vi "TLA_Picking List Get Table.vi"(8 "error in (no error)":errorcluster caption="错误输入（无错误）", 10 "JobNo":string, 11 "Traceability 引用句柄":refnum<k24>) -> (0 "error out":errorcluster caption="错误输出", 2 ".NET:System.Data.DataTable":T1 {"RemotingFormat" items=["Xml", "Binary"]}, 3 "Traceability 引用句柄输出":refnum<k24>)   [LabVIEW 2014, in "Traceability.lvlib"]
uses:
  D:/webservice/Traceability.dll
  Traceability.dll
  System.Data
  Traceability.lvlib
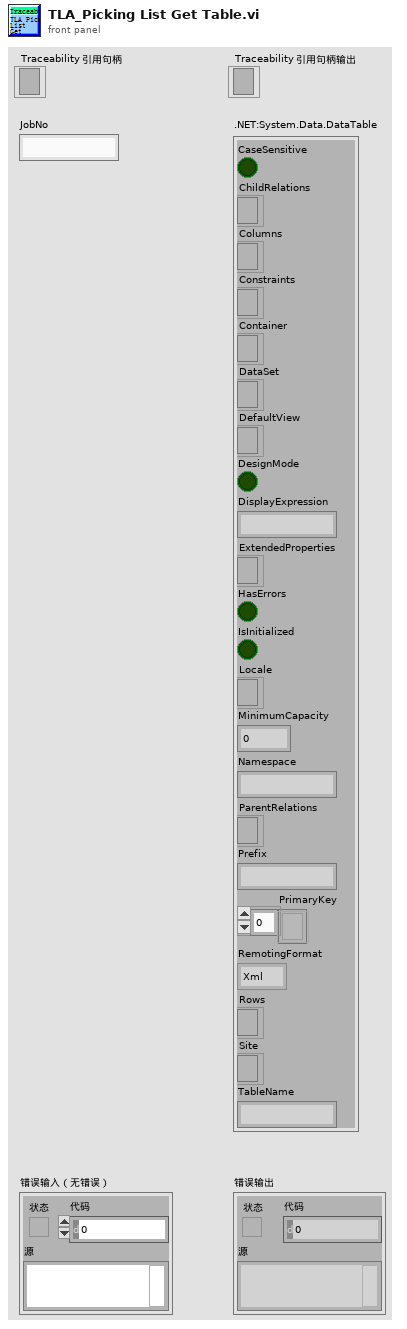
[diagram p1: front panel]
types:
  T1 = cluster{"CaseSensitive":bool, "ChildRelations":refnum<k24>, "Columns":refnum<k24>, "Constraints":refnum<k24>, "Container":refnum<k24>, "DataSet":refnum<k24>, "DefaultView":refnum<k24>, "DesignMode":bool, "DisplayExpression":string, "ExtendedProperties":refnum<k24>, "HasErrors":bool, "IsInitialized":bool, "Locale":refnum<k24>, "MinimumCapacity":i32, "Namespace":string, "ParentRelations":refnum<k24>, "Prefix":string, "PrimaryKey":refnum<k24>[], "RemotingFormat":i32, "Rows":refnum<k24>, "Site":refnum<k24>, "TableName":string}
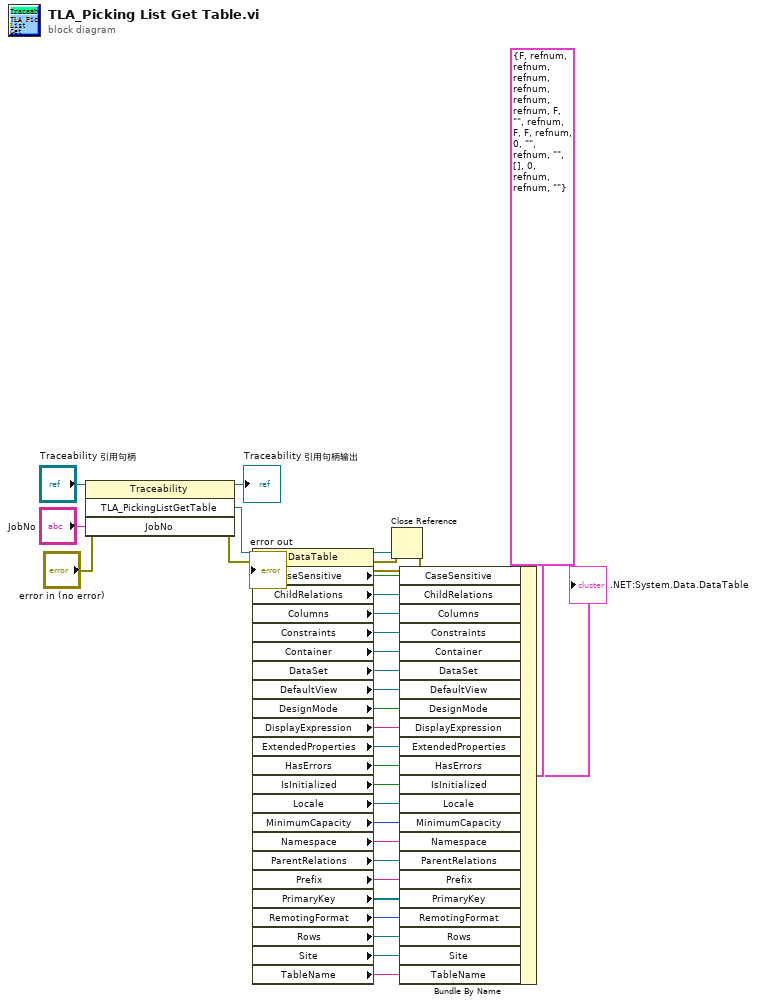
[diagram p0: block diagram]
diagram:
  n1 = invoke class="Traceability" method="TLA_PickingListGetTable"(reference="Traceability 引用句柄", error in="error in (no error)", "JobNo"="JobNo") -> (reference out=→"Traceability 引用句柄输出":refnum<k24>, error out=w4:errorcluster, "TLA_PickingListGetTable"=w30:refnum<k24>)  [unwired: 1 in, 1 out]
  n2 = property class="DataTable"(reference=w30, error in=w4) -> (reference out=w3:refnum<k24>, error out=w2:errorcluster, "CaseSensitive"=w27:bool, "ChildRelations"=w26:refnum<k24>, "Columns"=w25:refnum<k24>, "Constraints"=w24:refnum<k24>, "Container"=w23:refnum<k24>, "DataSet"=w22:refnum<k24>, "DefaultView"=w21:refnum<k24>, "DesignMode"=w20:bool, "DisplayExpression"=w19:string, "ExtendedProperties"=w18:refnum<k24>, "HasErrors"=w17:bool, "IsInitialized"=w16:bool, "Locale"=w15:refnum<k24>, "MinimumCapacity"=w14:i32, "Namespace"=w13:string, "ParentRelations"=w12:refnum<k24>, "Prefix"=w11:string, "PrimaryKey"=w10:refnum<k24>[], "RemotingFormat"=w9:i32, "Rows"=w8:refnum<k24>, "Site"=w7:refnum<k24>, "TableName"=w6:string)
  n3 = Close Reference(reference=w3, error in (no error)=w2) -> (error out=→"error out":errorcluster)
  n4 = Bundle By Name(cluster=T1 {"CaseSensitive"=FALSE, "ChildRelations"=refnum, "Columns"=refnum, "Constraints"=refnum, "Container"=refnum, "DataSet"=refnum, "DefaultView"=refnum, "DesignMode"=FALSE, "DisplayExpression"="", "ExtendedProperties"=refnum, "HasErrors"=FALSE, "IsInitialized"=FALSE, "Locale"=refnum, "MinimumCapacity"=0, "Namespace"="", "ParentRelations"=refnum, "Prefix"="", "PrimaryKey"=[], "RemotingFormat"=0, "Rows"=refnum, "Site"=refnum, "TableName"=""} (".NET:System.Data.DataTable"), "CaseSensitive"=w27, "ChildRelations"=w26, "Columns"=w25, "Constraints"=w24, "Container"=w23, "DataSet"=w22, "DefaultView"=w21, "DesignMode"=w20, "DisplayExpression"=w19, "ExtendedProperties"=w18, "HasErrors"=w17, "IsInitialized"=w16, "Locale"=w15, "MinimumCapacity"=w14, "Namespace"=w13, "ParentRelations"=w12, "Prefix"=w11, "PrimaryKey"=w10, "RemotingFormat"=w9, "Rows"=w8, "Site"=w7, "TableName"=w6) -> (→".NET:System.Data.DataTable":T1)
